vi "get stage name.vi"(8 "error in (no error)":errorcluster, 10 "stage_name":T1, 11 "id":i32) -> (0 "error out":errorcluster, 2 "stage_name out":T1, 3 "function return":i32)   [LabVIEW 2012, in "libximc.lvlib"]
doc: "result_t XIMC_API get_stage_name (device_t id, stage_name_t* stage_name);"
uses:
  libximc.lvlib
  libximc.dll
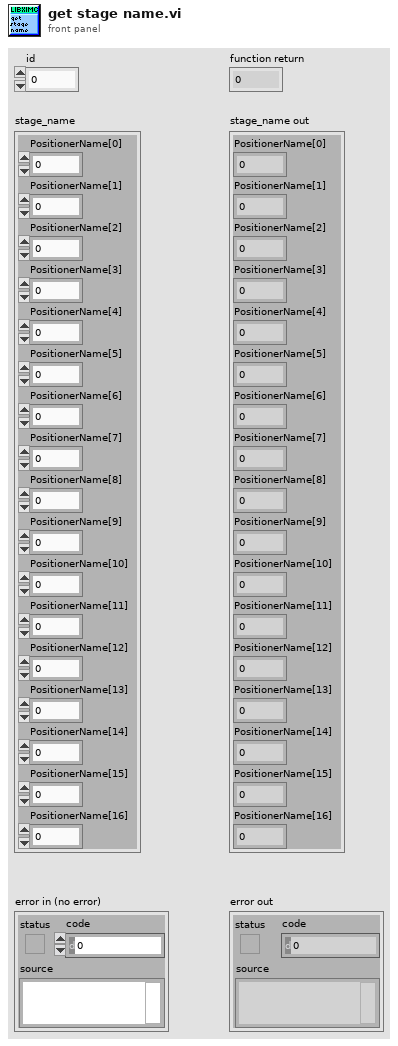
[diagram p1: front panel]
types:
  T1 = cluster{"PositionerName[0]":i8, "PositionerName[1]":i8, "PositionerName[2]":i8, "PositionerName[3]":i8, "PositionerName[4]":i8, "PositionerName[5]":i8, "PositionerName[6]":i8, "PositionerName[7]":i8, "PositionerName[8]":i8, "PositionerName[9]":i8, "PositionerName[10]":i8, "PositionerName[11]":i8, "PositionerName[12]":i8, "PositionerName[13]":i8, "PositionerName[14]":i8, "PositionerName[15]":i8, "PositionerName[16]":i8}
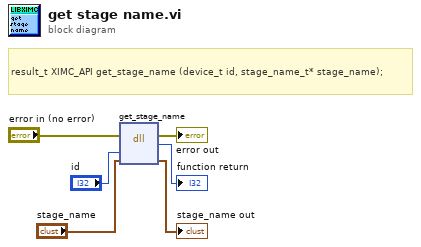
[diagram p0: block diagram]
diagram:
  # "result_t XIMC_API get_stage_name (device_t id, stage_name_t* stage_name);"
  n1 = dll-call lib="C:/Users/Stepan/Downloads/labview_2.9.11_testgen_thread/libximc.*" fn="get_stage_name"(error in="error in (no error)", "id"="id", "stage_name"="stage_name") -> (error out=→"error out":errorcluster, →"function return":i32, "stage_name"=→"stage_name out":T1)  [unwired: 3 in, 1 out]
